vi "testcolor.vi"() -> ()   [LabVIEW 2019]
panel:
  out "Image":T1(plugin-control)
  out "black":i32
  out "green":i32
  out "red":i32
  out "blue":i32
  out "yellow":i32
  out "Matches (Color Location 1)":T2(array[cluster]) {"Bounding Box"."y" format="%.2f"; "Bounding Box"."x" format="%.2f"; "Position"."y" format="%.2f"; "Position"."x" format="%.2f"; "Score" format="%.2f"; "Scale" format="%.2f"; "Angle" format="%.2f"}
  in  "Stop (F)":bool
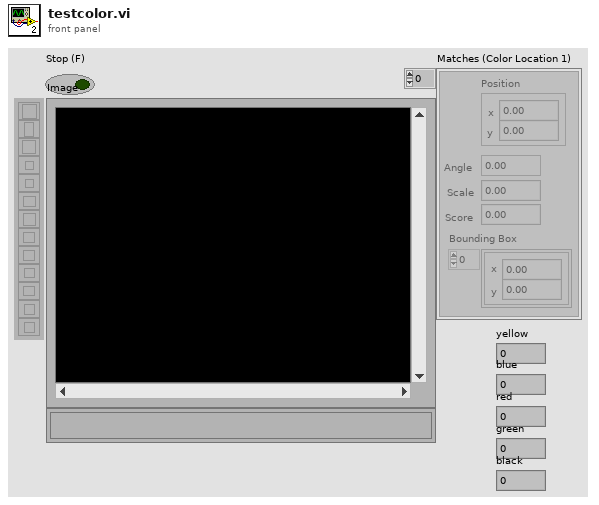
[diagram p1: front panel]
types:
  T1 = typedef "IMAQ Image.ctl" = refnum<image>
  T2 = cluster{"Position":cluster{"x":sgl, "y":sgl}, "Angle":sgl, "Scale":sgl, "Score":sgl, "Bounding Box":cluster{"x":sgl, "y":sgl}[]}[]
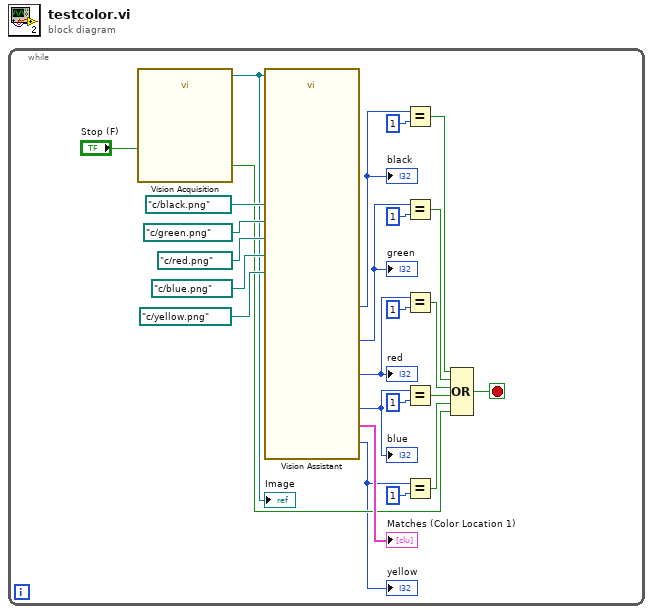
[diagram p0: block diagram]
diagram:
  n1 = while {
    stop <- w16 stop-if-true
    n2 = call "Vision Acquisition"("Stop (F)"="Stop (F)") -> ("Image Out"=w18:T1, "Stopped"=w17:bool)  [unwired: 24 in, 1 out]
    "Image" <- w18
    n3 = call "Vision Assistant"("Image In"=w18, "File Path (Color Location 1)"=path "c:/yellow.png", "File Path (Color Location 2)"=path "c:/blue.png", "File Path (Color Location 3)"=path "c:/red.png", "File Path (Color Location 4)"=path "c:/green.png", "File Path (Color Location 5)"=path "c:/black.png") -> ("Number of Matches (Color Location 5)"=w2:i32, "Number of Matches (Color Location 4)"=w1:i32, "Matches (Color Location 1)"=→"Matches (Color Location 1)":T2, "Number of Matches (Color Location 1)"=w4:i32, "Number of Matches (Color Location 2)"=w8:i32, "Number of Matches (Color Location 3)"=w10:i32)  [unwired: 10 in, 6 out]
    "red" <- w10
    "blue" <- w8
    "yellow" <- w4
    "green" <- w1
    "black" <- w2
    n4 = Equal?(x=w2, y=1) -> (x = y?=w13:bool)
    n5 = Equal?(x=w1, y=1) -> (x = y?=w12:bool)
    n6 = Equal?(x=w10, y=1) -> (x = y?=w6:bool)
    n7 = Equal?(x=w8, y=1) -> (x = y?=w7:bool)
    n8 = Equal?(x=w4, y=1) -> (x = y?=w3:bool)
    n9 = Compound Arithmetic op=OR(w13, w12, w6, w7, w3, w17) -> (w16:bool)
  }
